vi "RecursiveSynthApp.vi"() -> ()   [LabVIEW 2022 SP3]
uses:
  -AnnularRoutines/TransGeometry.ctl
  -AnnularRoutines/ArrayGeometry.ctl
panel:
  in  "Use Selected Files 2":bool
  in  "Listbox":i32[](listbox)
  in  "Filter Prams":T1={"low cutoff"=5, "order"=51, "high cutoff"=65}
  in  "Type of Mean":u16(ring)=4 items=["Mean from lines", "Mean just lines", "Poly Mean", "No mean", "Filter"]
  in  "Save Data":bool
  in  "Method":u16(ring) items=["Normal", "GPU", "ABUT", "EXPAND"]
  in  "Trans Geometry (mm)":T2={"Transducer"=0, "Geo Focus"=12.0, "a (radius)"=3.0, "# of rings"=5, "kerf space "=0.1, "Center Freq"=12.0} {"Transducer" items=["6D 12R 40 MHz"=0, "10D 31R 20 MHz"=1, "10D 23R 20 MHz"=2, "6D 23R 40 MHz"=3, "4.5D 10.7R 40 MHz"=4, "9D 23.5R 20 MHz"=5, "9D 25.8R 20MHz"=6, "Enter"=99]}
  in  "Use Selected Files":bool
  in  "Auto Select All?":bool
  in  "Save Center Elem?":bool
  in  "Save Sum?":bool
  in  "Save SF?":bool=TRUE
  in  "Root Directory":path
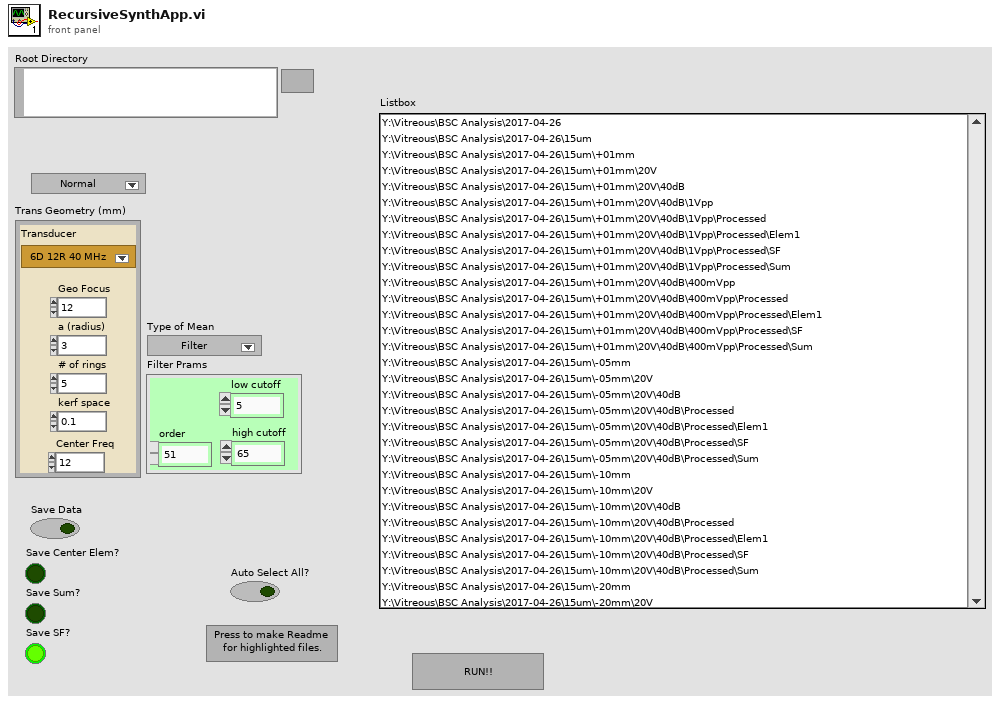
[diagram p1: front panel]
types:
  T1 = cluster{"low cutoff":i32, "order":i32, "high cutoff":i32}
  T2 = typedef "TransGeometry.ctl" = cluster{"Transducer":T3, "Geo Focus":dbl, "a (radius)":dbl, "# of rings":i32, "kerf space ":dbl, "Center Freq":dbl}
  T3 = typedef "ArrayGeometry.ctl" = u16
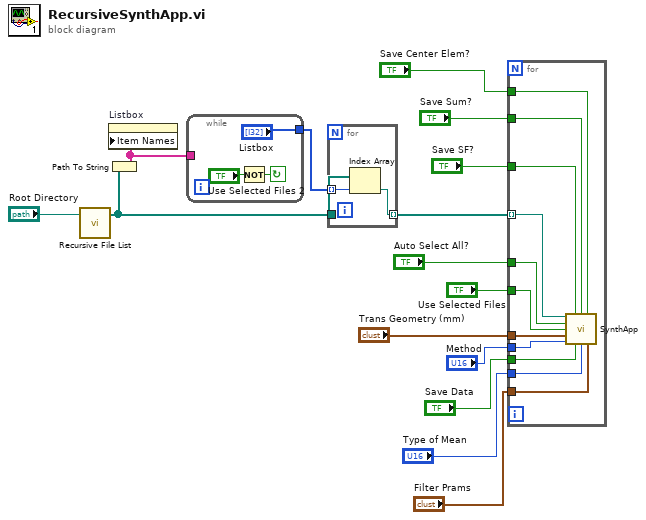
[diagram p0: block diagram]
diagram:
  n1 = call <vilib>:"Recursive File List.vi"("Folder Path"="Root Directory") -> ("All Folders"=w4:path[])  [unwired: 6 in, 4 out]
  n2 = Path To String(path=w4) -> (string=w1:string[])
  n3 = property on="Listbox" class="LstBox (strict)"("Item Names"=w1) -> ()  [unwired: 2 in, 2 out]
  n4 = while {
    tunnel: ["Listbox"] -> w2
    tunnel: w1 -> [_]
    stop <- w18 continue-if-true
    n5 = Not(x="Use Selected Files 2") -> (.not. x?=w18:bool)
  }
  n6 = for {
    tunnel: w4 -> [w21]
    tunnel: [w20] -> w3 mode=indexing
    tunnel: w2 -> [w19] mode=indexing
    n7 = Index Array(array=w21, index=w19) -> (element=w20:path)
  }
  n8 = for {
    tunnel: w3 -> [w32] mode=indexing
    tunnel: "Save SF?" -> [w31]
    tunnel: "Save Sum?" -> [w30]
    tunnel: "Save Center Elem?" -> [w29]
    tunnel: "Auto Select All?" -> [w28]
    tunnel: "Use Selected Files" -> [w27]
    tunnel: "Trans Geometry (mm)" -> [w26]
    tunnel: "Method" -> [w25]
    tunnel: "Save Data" -> [w24]
    tunnel: "Type of Mean" -> [w23]
    tunnel: "Filter Prams" -> [w22]
    n9 = call "SynthApp.vi"("Choose Directory"=w32, "Show SF?"=w31, "Show Sum?"=w30, "Save Center\nElem?"=w29, "Auto Select All?"=w28, "Use Selected Files"=w27, "Trans Geometry (mm)"=w26, "Method"=w25, "Save Data"=w24, "Type of Mean"=w23, "Filter Prams"=w22) -> ()  [unwired: 5 in]
  }
